vi "GaussianGlobal.vi"() -> ()   [LabVIEW 2011]
panel:
  in  "nLongSamples":i32
  in  "SD Estimate":dbl
  in  "SampleLength":string
  in  "MeasurementCenter":dbl
  in  "nPointsInRake":i32
  in  "FitStatus":string
  in  "nPointsSampled":i32
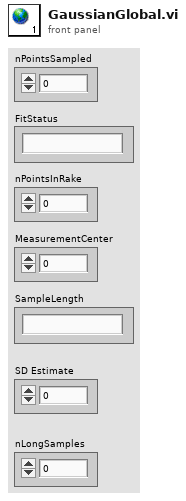
[diagram p1: front panel]
diagram:
